vi "FTW-Message-Interpret.vi"(0 "FTW Message":refnum<class "FTW-Message.lvclass">, 11 "error in":errorcluster) -> (4 "FTW Message out":refnum<class "FTW-Message.lvclass">, 6 "Sender Identity":string, 8 "Message Header":string, 10 "Message Body":string, 15 "error out":errorcluster)   [LabVIEW 2013, in "FTW-Message.lvclass"]
uses:
  FTW-Message.lvclass
panel:
  # "Inputs"
  # "Outputs"
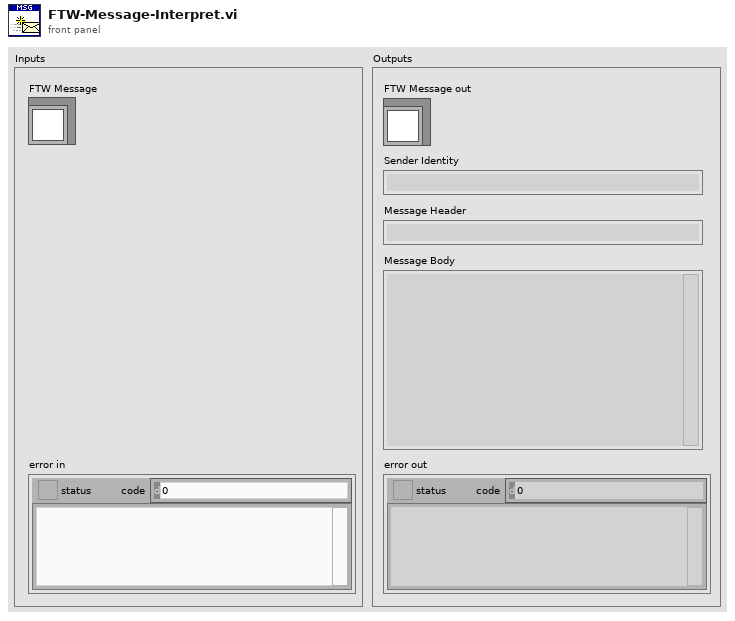
[diagram p1: front panel]
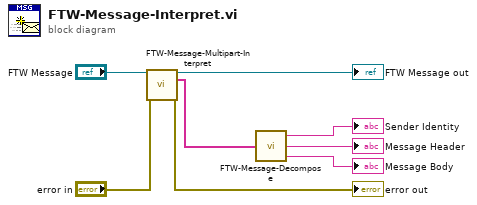
[diagram p0: block diagram]
diagram:
  n1 = call-dynamic "FTW-Message-Multipart-Interpret.vi"("FTW Message"="FTW Message", "error in"="error in") -> ("FTW Message out"=→"FTW Message out":refnum<class "FTW-Message.lvclass">, "Message Parts"=w4:string[], "error out"=→"error out":errorcluster)  [unwired: 11 in]
  n2 = call "FTW-Message-Decompose.vi"("Multipart Message"=w4) -> ("Sender Identity"=→"Sender Identity":string, "Message Header"=→"Message Header":string, "Message Body"=→"Message Body":string)  [unwired: 1 in]
